vi "SDF Small Gasifier RT - IO.vi"(0 "CIE Tags 2":T1, 1 "CIE Tags":T1) -> ()   [LabVIEW 2013]
uses:
  <userlib>/CIE/_TypeDefs/CIE Tags.ctl
  <userlib>/CIE/_TypeDefs/DBL CIE Tag.ctl
  <userlib>/CIE/_TypeDefs/BOOL CIE Tag.ctl
  <userlib>/CIE/_TypeDefs/I32 CIE Tag.ctl
  <userlib>/CIE/_TypeDefs/Enum CIE Tag.ctl
  <userlib>/CIE/_TypeDefs/STR CIE Tag.ctl
  <vilib>/NI/Current Value Table/DataTypes/Double_Read.vi
  <vilib>/NI/Current Value Table/DataTypes/String_Read.vi
  <vilib>/NI/Current Value Table/Type to Enum.vi
  <vilib>/NI/Current Value Table/DataTypes/Double_Type To Enum.vi
  <vilib>/NI/Current Value Table/DataTypes/String_Type To Enum.vi
  <vilib>/NI/Current Value Table/FGVs/CVT Globals.vi
  <vilib>/NI/Current Value Table/FGVs/Tag Memory.vi
  <vilib>/NI/Current Value Table/Memory Block.vi
  <vilib>/NI/Current Value Table/DataTypes/Double_Memory Block.vi
  <vilib>/NI/Current Value Table/DataTypes/String_Memory Block.vi
  <vilib>/NI/Current Value Table/Current Value Table.lvlib
panel:
  out "Numeric 2":dbl
  out "Missed Scan 2":bool
  out "Scan Error 2":errorcluster
  out "Missed Scan":bool
  out "Scan Error":errorcluster
  out "Value":string
  out "Numeric":dbl
  in  "Stop":bool
  out "Index":i32
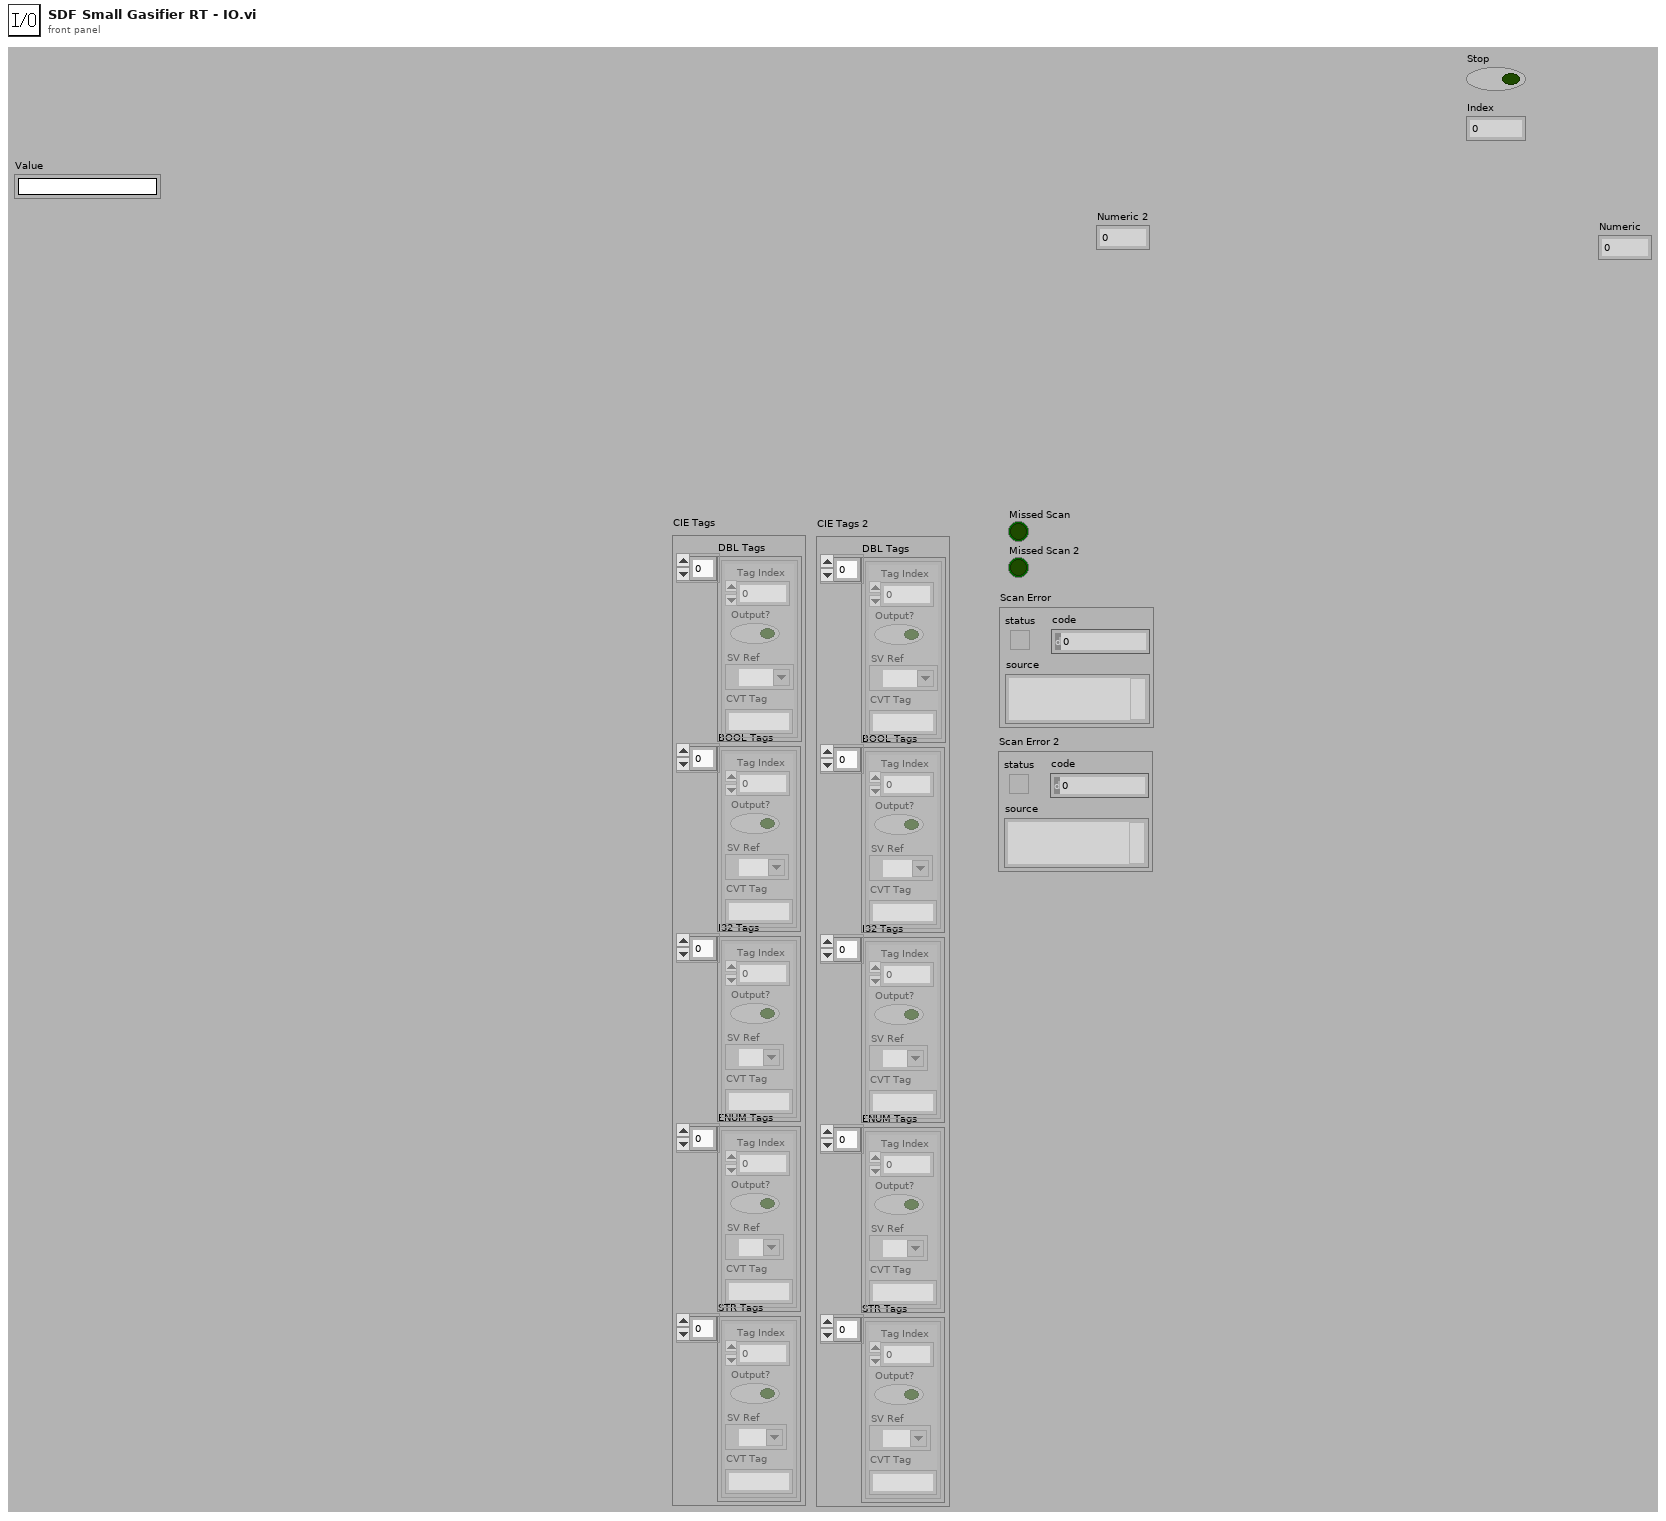
[diagram p1: front panel]
types:
  T1 = typedef "CIE Tags.ctl" = cluster{"DBL Tags":T2[], "BOOL Tags":T3[], "I32 Tags":T4[], "ENUM Tags":T5[], "STR Tags":T6[]}
  T2 = typedef "DBL CIE Tag.ctl" = cluster{"Tag Index":i32, "Output?":bool, "SV Ref":refnum<k21>, "CVT Tag":string}
  T3 = typedef "BOOL CIE Tag.ctl" = cluster{"Tag Index":i32, "Output?":bool, "SV Ref":refnum<k21>, "CVT Tag":string}
  T4 = typedef "I32 CIE Tag.ctl" = cluster{"Tag Index":i32, "Output?":bool, "SV Ref":refnum<k21>, "CVT Tag":string}
  T5 = typedef "Enum CIE Tag.ctl" = cluster{"Tag Index":i32, "Output?":bool, "SV Ref":refnum<k21>, "CVT Tag":string}
  T6 = typedef "STR CIE Tag.ctl" = cluster{"Tag Index":i32, "Output?":bool, "SV Ref":refnum<k21>, "CVT Tag":string}
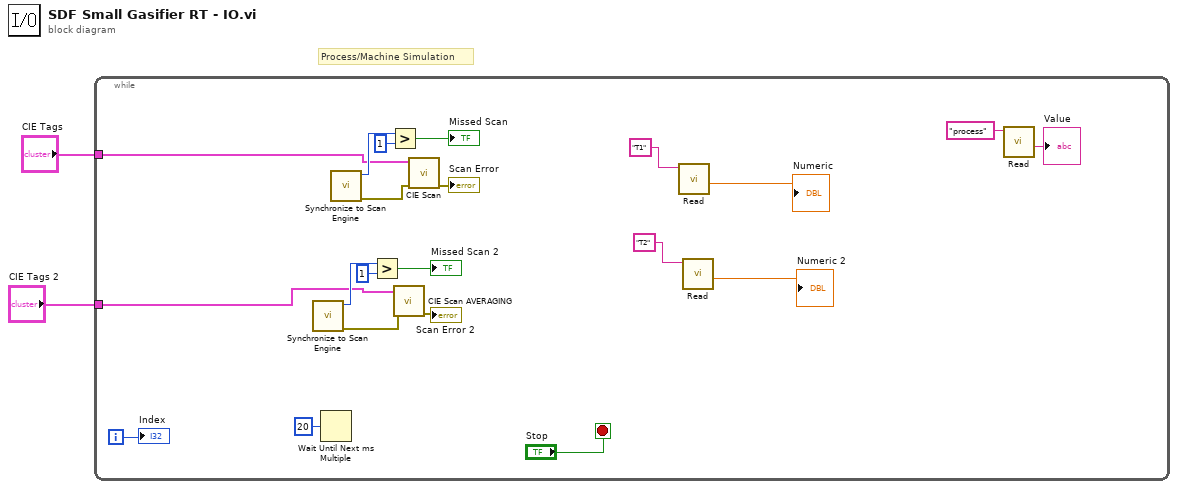
[diagram p0: block diagram]
diagram:
  # "Process/Machine Simulation"
  n1 = while {
    tunnel: "CIE Tags" -> [w12]
    tunnel: "CIE Tags 2" -> [w7]
    i -> [w22]
    stop <- "Stop" stop-if-true
    n2 = call <vilib>:"Synchronize to Scan Engine.vi"() -> ("error out"=w6:errorcluster, "scans since last call"=w8:u32)  [unwired: 10 in]
    n3 = Wait Until Next ms Multiple(millisecond multiple=u32 20) -> ()  [unwired: 1 out]
    n4 = call <vilib>:"Synchronize to Scan Engine.vi"() -> ("error out"=w13:errorcluster, "scans since last call"=w15:u32)  [unwired: 10 in]
    n5 = Greater?(x=w8, y=u32 1) -> (0:→"Missed Scan 2":bool)
    n6 = Greater?(x=w15, y=u32 1) -> (0:→"Missed Scan":bool)
    n7 = call <userlib>:"CIE Scan AVERAGING.vi"("error in (no error)"=w6, "CIE Tags"=w7) -> ("error put"=→"Scan Error 2":errorcluster)  [unwired: 9 in]
    n8 = call <userlib>:"CIE Scan.vi"("error in (no error)"=w13, "CIE Tags"=w12) -> ("error put"=→"Scan Error":errorcluster)  [unwired: 9 in]
    n9 = call-poly <vilib>:"Read.vi"("Tag Name"="T1") -> ("Value"=→"Numeric":dbl)  [unwired: 9 in, 1 out]
    n10 = call-poly <vilib>:"Read.vi"("Tag Name"="T2") -> ("Value"=→"Numeric 2":dbl)  [unwired: 9 in, 1 out]
    n11 = call-poly <vilib>:"Read.vi"("Tag Name"="process") -> ("Value"=→"Value":string)  [unwired: 9 in, 1 out]
    "Index" <- w22
  }
